vi "Self-Test.vi"(0 "VISA resource name":refnum<visa-resource-name>, 11 "error in (no error)":errorcluster) -> (4 "VISA resource name out":refnum<visa-resource-name>, 6 "Self-Test Result Code":i32, 15 "error out":errorcluster)   [LabVIEW 2012, in "NH Research Regenerative Test Series.lvlib"]
doc: "Causes the module to reset all channels and run a self test. All errors are cleared if possible except those generated during self test. This command will generate PROM, Firmware, Configuration and Calibration Errors as required. If there is no Calibration Error, calibration data of the specific channel is copied from FLASH to RAM and used. Returns a 0 if no errors, a 1 if any errors."
uses:
  <instrlib>/NH Research Regenerative Test Series/NH Research Regenerative Test Series.lvlib
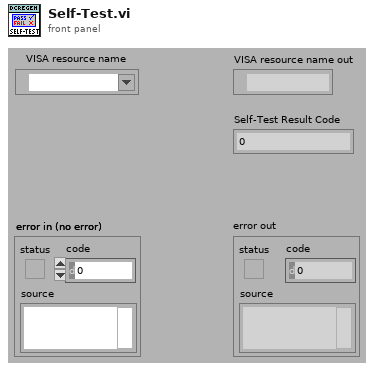
[diagram p1: front panel]
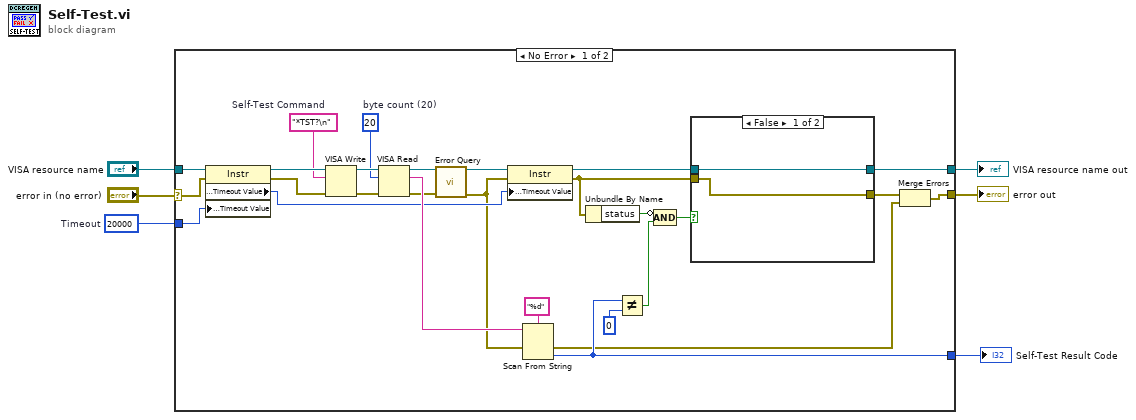
[diagram p0: block diagram]
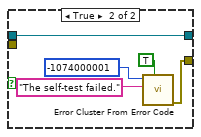
[diagram p2: hidden frame]
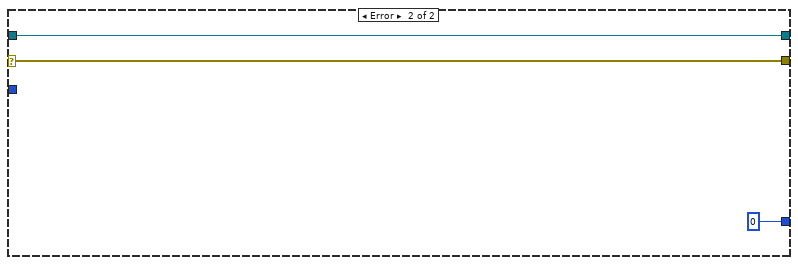
[diagram p3: hidden frame]
diagram:
  w3 = u32 20000  # Timeout
  n1 = case shown="No Error" "error in (no error)" {
    selector: "error in (no error)" -> [w15 w42]
    tunnel: "VISA resource name" -> [w30 w43]
    tunnel: [w11 w43] -> w5
    tunnel: [w12 w42] -> w4
    tunnel: w3 -> [w27 _]
    tunnel: [w17 0] -> w2
    frame No Error {
      w29 = u32 20  # byte count (20)
      w23 = "*TST?\n"  # Self-Test Command
      n2 = property on="Property Node" class="Instr"(reference=w30, error in=w15, "General Settings:Timeout Value"=w27) -> (reference out=w25:refnum<visa-resource-name>, error out=w26:errorcluster, "General Settings:Timeout Value"=w24:u32)
      n3 = VISA Write(VISA resource name=w25, write buffer=w23, error in (no error)=w26) -> (VISA resource name out=w32:refnum<visa-resource-name>, error out=w31:errorcluster)  [unwired: 1 out]
      n4 = VISA Read(VISA resource name=w32, byte count=w29, error in (no error)=w31) -> (VISA resource name out=w10:refnum<visa-resource-name>, read buffer=w28:string, error out=w9:errorcluster)  [unwired: 1 out]
      n5 = call <instrlib>:"Error Query.vi"("VISA resource name"=w10, "error in (no error)"=w9) -> ("VISA resource name out"=w8:refnum<visa-resource-name>, "error out"=w7:errorcluster)  [unwired: 10 in, 2 out]
      n6 = property on="Property Node" class="Instr"(reference=w8, error in=w7, "General Settings:Timeout Value"=w24) -> (reference out=w22:refnum<visa-resource-name>, error out=w21:errorcluster)
      n7 = Scan From String(format string="%d", input string=w28, error in=w7) -> (error out=w13:errorcluster, output 1=w17:i32)  [unwired: 2 in, 2 out]
      n8 = Unbundle By Name(w21) -> ("status"=w19:bool)
      n9 = Not Equal?(x=w17, y=0) -> (x != y?=w20:bool)
      n10 = Compound Arithmetic op=AND(invert w19, w20) -> (w18:bool)
      n11 = case shown="False" w18 {
        tunnel: w22 -> [w35 w40]
        tunnel: w21 -> [w34 _]
        tunnel: [w34 w36] -> w14
        tunnel: [w35 w40] -> w11
        frame False {
        }
        frame True {
          n12 = call <vilib>:"Error Cluster From Error Code.vi"("show call chain? (False)"=TRUE, "error message (\"\")"="The self-test failed." ("Source (VI Name)"), "error code (0)"=-1074000001 ("Code")) -> ("error out"=w36:errorcluster)  [unwired: 6 in]
        }
      }
      n13 = Merge Errors(w14, w13) -> (w12:errorcluster)
    }
    frame Error {
    }
  }
  "Self-Test Result Code" <- w2
  "VISA resource name out" <- w5
  "error out" <- w4
